vi "4 Helper - apply max slew rate.vi"(10 "Maximum Slew Rate (#/s)":dbl=1.0, 11 "Control Value In":dbl) -> (3 "Control Value Out":dbl)   [LabVIEW 2011]
doc: "applies a maximum slew rate to the input signal."
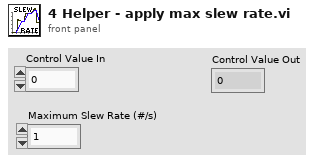
[diagram p1: front panel]
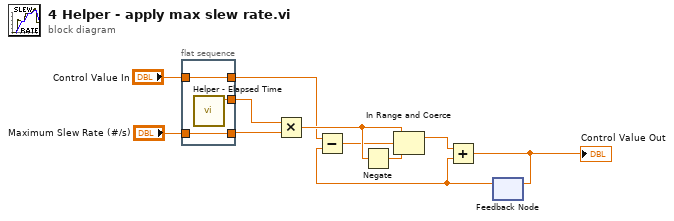
[diagram p0: block diagram]
diagram:
  n1 = flat-sequence {
    tunnel: [w14] -> w9
    tunnel: "Maximum Slew Rate (#/s)" -> [w13]
    tunnel: [w13] -> w11
    tunnel: [w12] -> w2
    tunnel: "Control Value In" -> [w12]
    frame #0 {
      n2 = call "Helper - Elapsed Time.vi"() -> ("Time Elapsed (s)\nSince Last Iteration"=w14:dbl)  [unwired: 10 in, 1 out]
    }
  }
  n3 = Multiply(x=w9, y=w11) -> (x*y=w6:dbl)
  n4 = Negate(x=w6) -> (-x=w5:dbl)
  n5 = feedback #1() -> (w8:dbl)  [unwired: 1 in]
  n6 = Subtract(x=w2, y=w8) -> (x-y=w4:dbl)
  n7 = In Range and Coerce(upper limit=w6, x=w4, lower limit=w5) -> (coerced(x)=w7:dbl)  [unwired: 1 out]
  n8 = Add(x=w7, y=w8) -> (x+y=w3:dbl)
  "Control Value Out" <- w3
  n9 = feedback-in #1(w3) -> ()
